vi "Battery Percentage (SubVI).vi"(9 "Battery Voltage":dbl, 10 "Min Battery Voltage":dbl, 11 "Max Battery Voltage":dbl) -> (3 "Battery Percent Remaining":dbl)   [LabVIEW 2013]
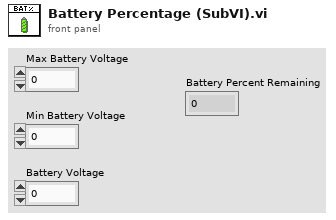
[diagram p1: front panel]
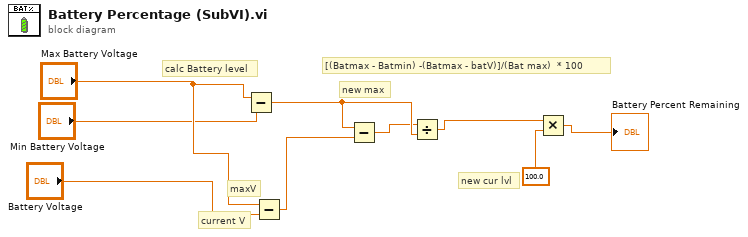
[diagram p0: block diagram]
diagram:
  # "new cur lvl"
  # "new max"
  # "current V"
  # "maxV"
  # "[(Batmax - Batmin) -(Batmax - batV)]/(Bat max)  * 100"
  # "calc Battery level"
  n1 = Subtract(x="Max Battery Voltage", y="Min Battery Voltage") -> (x-y=w6:dbl)
  n2 = Subtract(x="Max Battery Voltage", y="Battery Voltage") -> (x-y=w3:dbl)
  n3 = Subtract(x=w6, y=w3) -> (x-y=w5:dbl)
  n4 = Divide(x=w5, y=w6) -> (x/y=w7:dbl)
  n5 = Multiply(x=w7, y=100.0) -> (x*y=→"Battery Percent Remaining":dbl)
